vi "Start Calibrate TxPwr Dll.vi"(0 "CART TCP Connection In":refnum<k5>, 1 "TxPwrCalFreq":i32, 5 "Need Send Cal Command":u8, 7 "isFirstFreq":u8, 9 "TxPwrCalGain":u32, 11 "TxPwrCalRate":string, 12 "TxPwrCalCh":u32) -> (4 "CART TCP Connection Out":refnum<k5>, 6 "Need More Pwr Reporting":i16, 8 "StatusIsFalse":i16)   [LabVIEW 2012]
uses:
  WLAN/UUT/QCA/Controls/QCA NART Response Type.ctl
  WLAN/UUT/QCA/Controls/QCA NART Response SubType.ctl
panel:
  out "Messages Logged":string[](array[string])
  in  "error in (no error)":errorcluster
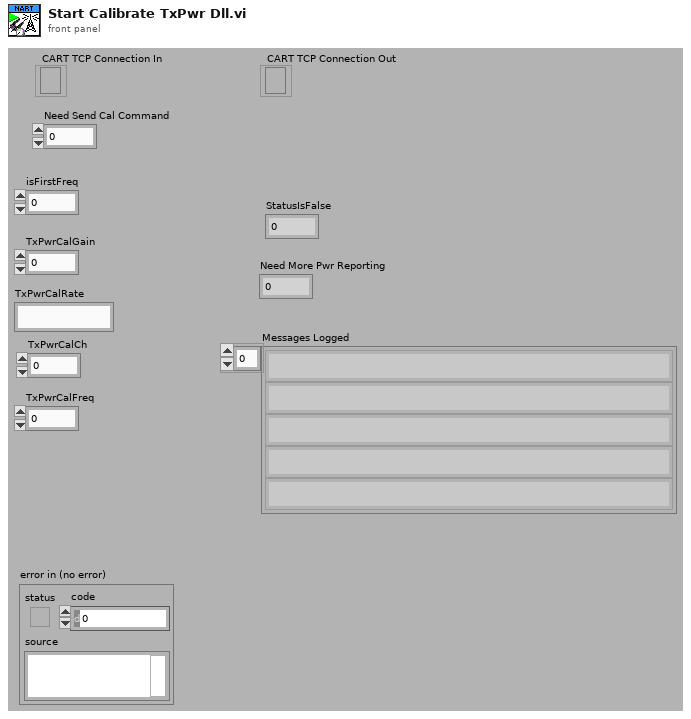
[diagram p1: front panel]
types:
  T1 = typedef "QCA NART Response Type.ctl" = enum16{"DEBUG", "CONTROL", "INFO", "WARNING", "ERROR", "NONE"}
  T2 = typedef "QCA NART Response SubType.ctl" = enum16{"NONE", "OK", "ON", "OFF", "BEGIN", "DONE"}
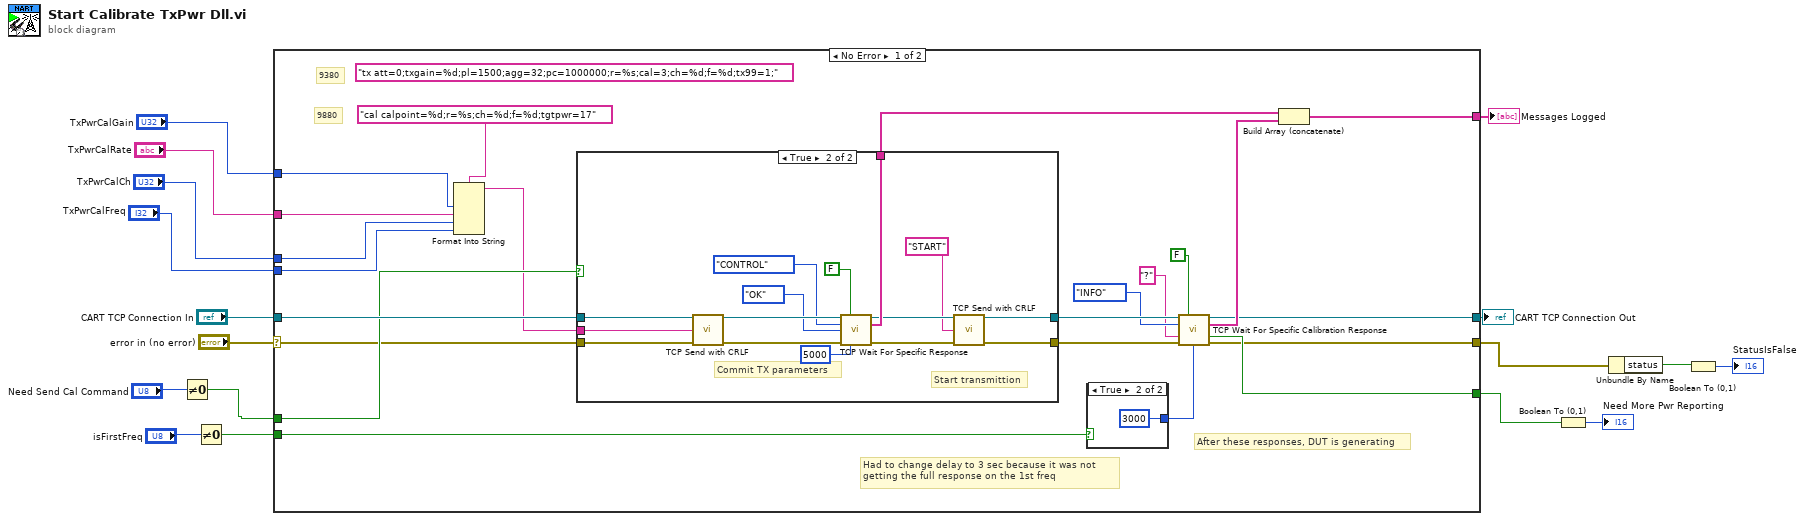
[diagram p0: block diagram]
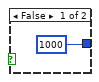
[diagram p2: hidden frame]
diagram:
  n1 = Not Equal To 0?(x="Need Send Cal Command") -> (x != 0?=w5:bool)
  n2 = Not Equal To 0?(x="isFirstFreq") -> (x != 0?=w3:bool)
  n3 = case shown="No Error" "error in (no error)" {
    selector: "error in (no error)" -> [w25 w60]
    tunnel: [w28 w60] -> w13
    tunnel: "CART TCP Connection In" -> [w39 w59]
    tunnel: [w29 w59] -> w15
    tunnel: [w36 _] -> w14
    tunnel: [w31 _] -> w1
    tunnel: w5 -> [w27 _]
    tunnel: w3 -> [w24 _]
    tunnel: "TxPwrCalGain" -> [w23 _]
    tunnel: "TxPwrCalRate" -> [w22 _]
    tunnel: "TxPwrCalCh" -> [w21 _]
    tunnel: "TxPwrCalFreq" -> [w20 _]
    frame No Error {
      (unwired) "tx att=0;txgain=%d;pl=1500;agg=32;pc=1000000;r=%s;cal=3;ch=%d;f=%d;tx99=1;" ("Name")
      # "9380"
      # "9880"
      # "Had to change delay to 3 sec because it was not \ngetting the full response on the 1st freq"
      # "After these responses, DUT is generating"
      n4 = Format Into String(format string="cal calpoint=%d;r=%s;ch=%d;f=%d;tgtpwr=17" ("Name"), w23, w22, w21, w20) -> (resulting string=w19:string)  [unwired: 2 in, 1 out]
      n5 = case shown="True" w27 {
        tunnel: w39 -> [w43 w58]
        tunnel: [_ w56] -> w38
        tunnel: [w43 w51] -> w35
        tunnel: [w42 w50] -> w34
        tunnel: w25 -> [w42 w47]
        tunnel: w19 -> [_ w46]
        frame False {
        }
        frame True {
          # "Start transmittion"
          # "Commit TX parameters"
          n6 = call "TCP Send with CRLF.vi"("CART TCP Connection"=w58, "data in"=w46, "error IO"=w47) -> ("CART TCP Connection Out"=w55:refnum<k5>, "error out"=w54:errorcluster)  [unwired: 11 in]
          n7 = call "TCP Wait For Specific Response.vi"("TCP Connection In"=w55, "Next response (t)"=FALSE, "Expected Type"=QCA_NART_Response_Type."CONTROL", "Expected Subtype (none)"=QCA_NART_Response_SubType."OK", "error in"=w54, "Timeout (250 ms)"=5000 ("Timeout (100ms)")) -> ("TCP Connection Out"=w52:refnum<k5>, "TCP Messages"=w56:string[], "error out"=w53:errorcluster)  [unwired: 6 in, 1 out]
          n8 = call "TCP Send with CRLF.vi"("CART TCP Connection"=w52, "data in"="START" ("Expected Message Start (\"\":any)"), "error IO"=w53) -> ("CART TCP Connection Out"=w51:refnum<k5>, "error out"=w50:errorcluster)  [unwired: 11 in]
        }
      }
      n9 = case shown="True" w24 {
        tunnel: [1000 ("Timeout (250 ms)") 3000 ("Timeout (250 ms)")] -> w32
        frame False {
        }
        frame True {
        }
      }
      n10 = call "TCP Wait For Specific Calibration Response.vi"("TCP Connection In"=w35, "Next response (t)"=FALSE, "Expected Type"=QCA_NART_Response_Type."INFO", "Expected Message Start (\"\":any)"="?" ("Expected Message Start (\"\":any)"), "error in"=w34, "Timeout (250 ms)"=w32) -> ("TCP Connection Out"=w29:refnum<k5>, "TCP Messages"=w37:string[], "More Pwr Reporting?"=w31:bool, "error out"=w28:errorcluster)  [unwired: 5 in, 1 out]
      n11 = Build Array (concatenate)(w38, w37) -> (w36:string[])
    }
    frame Error {
    }
  }
  "CART TCP Connection Out" <- w15
  "Messages Logged" <- w14
  n12 = Boolean To (0,1)(Boolean=w1) -> (0, 1=→"Need More Pwr Reporting":i16)
  n13 = Unbundle By Name(w13) -> ("status"=w11:bool)
  n14 = Boolean To (0,1)(Boolean=w11) -> (0, 1=→"StatusIsFalse":i16)
